vi "Doc_VI_Group_Name.vi"(9 "Group Name is second\npart of file name":bool, 11 "FileName":string) -> (3 "Section Name":string)   [LabVIEW 2019]
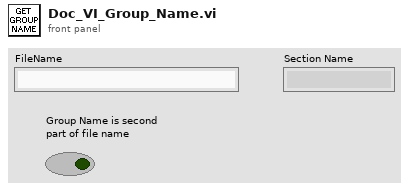
[diagram p1: front panel]
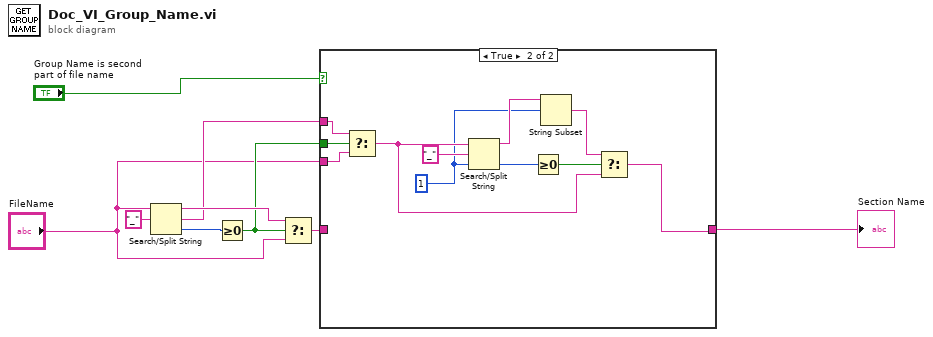
[diagram p0: block diagram]
diagram:
  n1 = Search/Split String(string="FileName", search string/char (-)="_") -> (substring before match=w7:string, match + rest of string=w6:string, offset of match=w9:i32)  [unwired: 1 in]
  n2 = Greater Or Equal To 0?(x=w9) -> (x >= 0?=w5:bool)
  n3 = Select(t=w7, s=w5, f="FileName") -> (s? t:f=w2:string)
  n4 = case shown="True" "Group Name is second\npart of file name" {
    tunnel: w6 -> [_ w21]
    tunnel: w5 -> [_ w20]
    tunnel: "FileName" -> [_ w19]
    tunnel: w2 -> [w10 _]
    tunnel: [w10 w15] -> w1
    frame False {
    }
    frame True {
      w12 = 1 ("offset (0)")
      n5 = Select(t=w21, s=w20, f=w19) -> (s? t:f=w14:string)
      n6 = Search/Split String(string=w14, search string/char (-)="_", offset (0)=w12) -> (substring before match=w13:string, offset of match=w16:i32)  [unwired: 1 out]
      n7 = Greater Or Equal To 0?(x=w16) -> (x >= 0?=w17:bool)
      n8 = String Subset(string=w13, offset (0)=w12) -> (substring=w11:string)  [unwired: 1 in]
      n9 = Select(t=w11, s=w17, f=w14) -> (s? t:f=w15:string)
    }
  }
  "Section Name" <- w1
